vi "Stage1V3_0921.vi"(6 "Center Point":sgl[](array[numeric]), 8 "error in (no error)":errorcluster, 10 "XYData":sgl[][](array[numeric]) format="%#_5p", 11 "Application ref in":refnum<vi>) -> ()   [LabVIEW 2020]
panel:
  out "Center Point re":sgl[](array[numeric])
  out "img1":sgl[][](array[numeric])
  out "output array":sgl[][](array[numeric])
  in  "XYData 2":sgl[][](array[numeric]) format="%#_5p"
  in  "path":string="3.6"
  in  "Python version 2":string="3.6"
  in  "module path 2":path=path "D:/Git repo/pythonProject/STM_Python_Modules/util.py"
  out "Error out":errorcluster
  out "XY":sgl[][](array[numeric])
  out "WH":sgl[][](array[numeric])
  in  "Array":sgl[](array[numeric])
  in  "Python version":string="3.6"
  in  "module path":path=path "D:/Git repo/pythonProject/STM_Python_Modules/ObjDet.py"
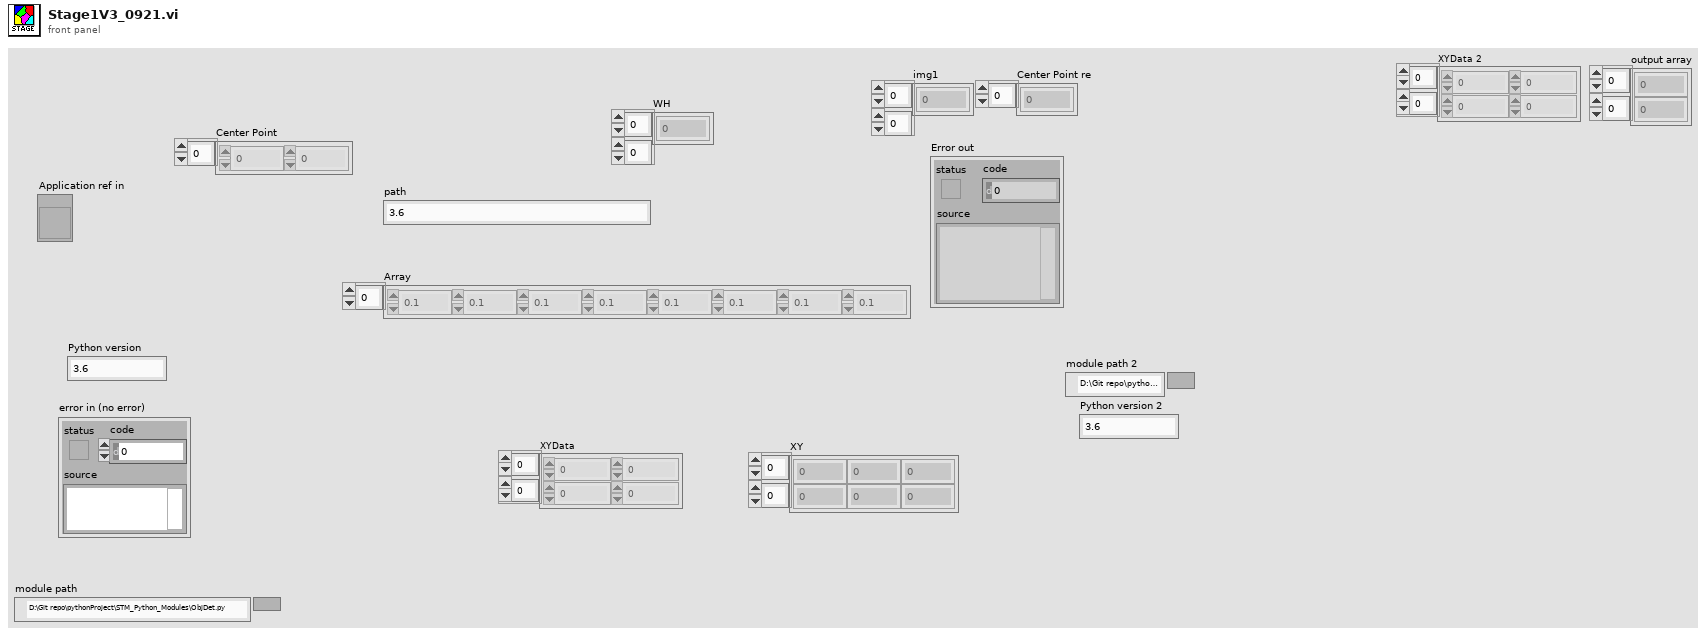
[diagram p1: front panel]
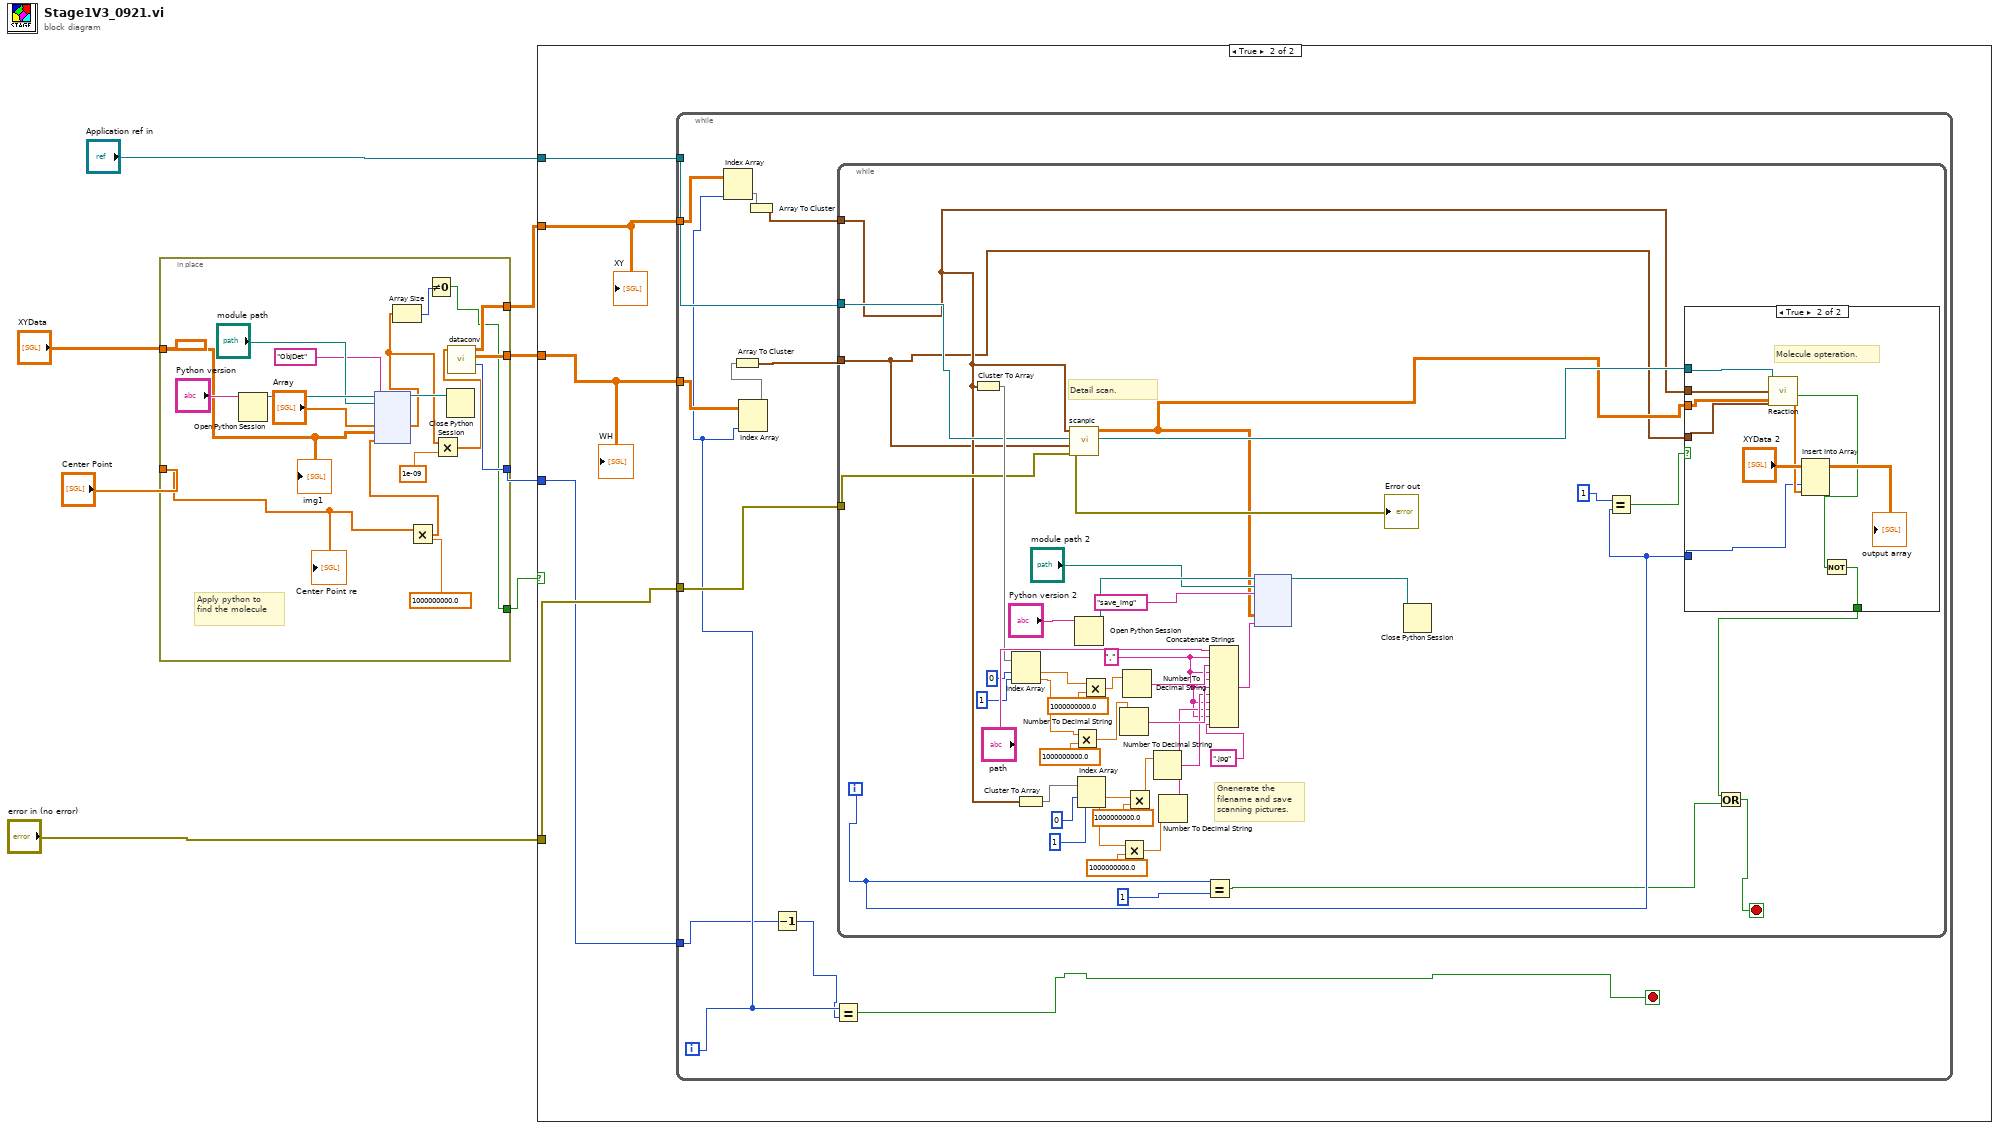
[diagram p0: block diagram]
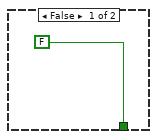
[diagram p3: hidden frame]
diagram:
  n1 = in-place {
    in-place-border: "XYData" -> [w18]
    in-place-border: [w26] -> w6
    in-place-border: [w25] -> w4
    in-place-border: [w24] -> w3
    in-place-border: "Center Point" -> [w15]
    in-place-border: [w9] -> w1
    # "Apply python to find the molecule"
    n2 = Open Python Session(python version="Python version") -> (session out=w23:refnum<k35>)  [unwired: 2 in, 1 out]
    n3 = Multiply(x=w15, y=1000000000.0) -> (x*y=w14:dbl[])
    n4 = node(w23, "module path", "ObjDet" ("function name"), "Array", w18, w14) -> (w22:refnum<k35>, w12:sgl[])  [unwired: 3 in, 3 out]
    n5 = Array Size(array=w12) -> (size(s)=w10:i32)
    n6 = Not Equal To 0?(x=w10) -> (x != 0?=w9:bool)
    n7 = Multiply(x=w12, y=1e-09) -> (x*y=w11:dbl[])
    n8 = Close Python Session(session in=w22) -> ()  [unwired: 1 in, 1 out]
    n9 = call "dataconv.vi"("Array"=w11) -> ("n"=w26:i32, "WH"=w24:sgl[][], "XY"=w25:sgl[][])  [unwired: 8 in]
    "img1" <- w18
    "Center Point re" <- w15
  }
  n10 = case shown="True" w1 {
    tunnel: "Application ref in" -> [_ w31]
    tunnel: "error in (no error)" -> [_ w30]
    tunnel: w6 -> [_ w29]
    tunnel: w4 -> [_ w28]
    tunnel: w3 -> [_ w27]
    frame False {
    }
    frame True {
      n11 = while {
        tunnel: w31 -> [w43]
        tunnel: w30 -> [w42]
        tunnel: w29 -> [w33]
        tunnel: w28 -> [w41]
        tunnel: w27 -> [w38]
        i -> [w35]
        stop <- w34 stop-if-true
        n12 = Index Array(array=w41, index (col)=w35) -> (element=w40:sgl[])  [unwired: 1 in]
        n13 = Index Array(array=w38, index (col)=w35) -> (element=w37:sgl[])  [unwired: 1 in]
        n14 = Array To Cluster(array=w37) -> (cluster=w36:cluster{"WH[0]":sgl, "WH[1]":sgl})
        n15 = Array To Cluster(array=w40) -> (cluster=w39:cluster{"XY[0]":sgl, "XY[1]":sgl})
        n16 = Decrement(x=w33) -> (x-1=w32:i32)
        n17 = Equal?(x=w35, y=w32) -> (x = y?=w34:bool)
        n18 = while {
          tunnel: w39 -> [w48]
          tunnel: w36 -> [w47]
          tunnel: w43 -> [w55]
          tunnel: w42 -> [w54]
          i -> [w51]
          stop <- w44 stop-if-true
          w70 = "," ("string")
          # "Gnenerate the filename and save scanning pictures."
          # "Detail scan."
          n19 = Cluster To Array(cluster=w48) -> (array=w80:sgl[])
          n20 = Index Array(array=w80, index #1=0 ("index"), index #2=1) -> (element #1=w57:sgl, element #2=w59:sgl)
          n21 = Cluster To Array(cluster=w48) -> (array=w73:sgl[])
          n22 = call "scanpic.vi"("error in (no error)"=w54, "Size (m)"=w47, "Application ref in"=w55, "Center coordinates (m)"=w48) -> ("Error out"=→"Error out":errorcluster, "Application ref out"=w53:refnum<vi>, "Data"=w52:sgl[][])  [unwired: 5 in]
          n23 = Multiply(x=w59, y=1000000000.0) -> (x*y=w58:dbl)
          n24 = Open Python Session(python version="Python version 2") -> (session out=w86:refnum<k35>)  [unwired: 2 in, 1 out]
          n25 = Index Array(array=w73, index #1=0 ("index"), index #2=1) -> (element #1=w61:sgl, element #2=w63:sgl)
          n26 = Multiply(x=w57, y=1000000000.0) -> (x*y=w56:dbl)
          n27 = Number To Decimal String(number=w58) -> (decimal integer string=w76:string)  [unwired: 1 in]
          n28 = Multiply(x=w63, y=1000000000.0) -> (x*y=w62:dbl)
          n29 = Number To Decimal String(number=w56) -> (decimal integer string=w78:string)  [unwired: 1 in]
          n30 = Multiply(x=w61, y=1000000000.0) -> (x*y=w60:dbl)
          n31 = Number To Decimal String(number=w60) -> (decimal integer string=w72:string)  [unwired: 1 in]
          n32 = Number To Decimal String(number=w62) -> (decimal integer string=w71:string)  [unwired: 1 in]
          n33 = Equal?(x=w51, y=1) -> (x = y?=w46:bool)
          n34 = Concatenate Strings("path", w70, w78, w70, w76, w70, w72, w70, w71, w70, ".jpg" ("string")) -> (w68:string)
          n35 = node(w86, "module path 2", "save_img" ("function name"), w52, w68) -> (w85:refnum<k35>)  [unwired: 5 in, 3 out]
          n36 = Close Python Session(session in=w85) -> ()  [unwired: 1 in, 1 out]
          n37 = Equal?(x=1, y=w51) -> (x = y?=w49:bool)
          n38 = case shown="True" w49 {
            tunnel: w53 -> [_ w96]
            tunnel: w48 -> [_ w95]
            tunnel: w47 -> [_ w94]
            tunnel: w51 -> [_ w93]
            tunnel: w52 -> [_ w92]
            tunnel: [FALSE w90] -> w45
            frame False {
            }
            frame True {
              # "Molecule opteration."
              n39 = call "Reaction.vi"("Size (m)"=w94, "Center coordinates (m)"=w95, "XYData"=w92, "Application ref in"=w96) -> ("rollout"=w98:dbl[], "Boolean"=w91:bool)  [unwired: 4 in, 2 out]
              n40 = Insert Into Array(array="XYData 2", index (col)=w93, new element=w98) -> (→"output array":sgl[][])  [unwired: 1 in]
              n41 = Not(x=w91) -> (.not. x?=w90:bool)
            }
          }
          n42 = Or(x=w45, y=w46) -> (x .or. y?=w44:bool)
        }
      }
      "WH" <- w27
      "XY" <- w28
    }
  }
